vi "GlobalDataNames.vi"() -> ()   [LabVIEW 2015]
panel:
  in  "DataNames":string[](array[string])
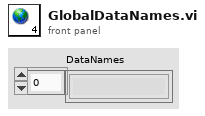
[diagram p1: front panel]
diagram:
